vi "Initialise_scan_mirror_positions.vi"(8 "error in (no error)":errorcluster) -> (0 "error out":errorcluster)   [LabVIEW 2012]
uses:
  Custom Controls/scan mode main settings tab.ctl
  GFG/GFGbooleanGet.vi
  <vilib>/DAQmx/create/channels.llb/DAQmx Create Channel (AO-Voltage-Basic).vi
  <vilib>/DAQmx/write.llb/DAQmx Write.vi
  <vilib>/DAQmx/write.llb/DAQmx Write (Analog 1D DBL NChan 1Samp).vi
  GFG/GFGstringGet.vi
  GFG/GFG library.lvlib
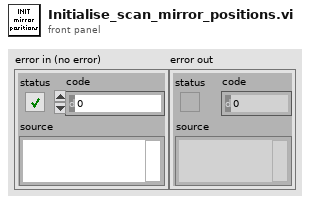
[diagram p1: front panel]
types:
  T1 = typedef "scan mode main settings tab.ctl" = enum32{"2D frame", "2D line scan", "general settings", "Z Stack", "piezo"}
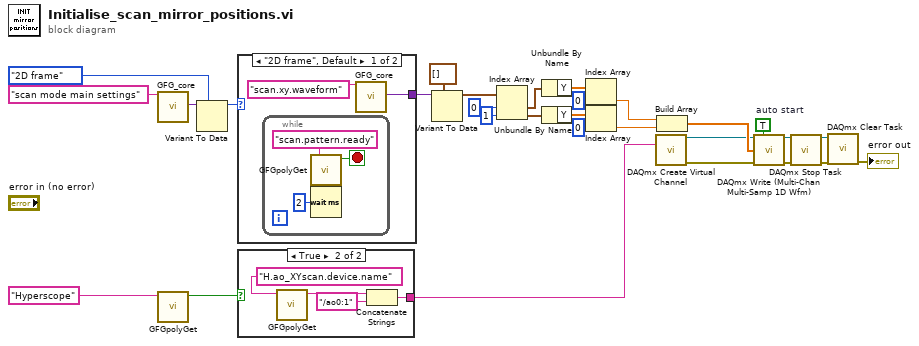
[diagram p0: block diagram]
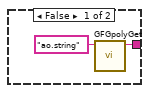
[diagram p2: hidden frame]
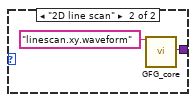
[diagram p3: hidden frame]
diagram:
  w6 = TRUE  # auto start
  n1 = call "GFG_core.vi"("Variable Name in"="scan mode main settings") -> ("Variant Out"=w28:variant)  [unwired: 12 in, 6 out]
  n2 = call-poly "GFGpolyGet.vi"("Variable Name in"="Hyperscope") -> ("Boolean Value OUT"=w13:bool)  [unwired: 9 in, 1 out]
  n3 = Variant To Data(type=scan_mode_main_settings_tab."2D frame" ("scan mode main settings"), Variant=w28) -> (data=w26:T1)  [unwired: 1 in, 1 out]
  n4 = case shown="\"2D frame\", Default" w26 {
    tunnel: [w30 w35] -> w29
    frame "2D frame", Default {
      n5 = while {
        stop <- w33 stop-if-true
        n6 = call-poly "GFGpolyGet.vi"("Variable Name in"="scan.pattern.ready") -> ("Boolean Value OUT"=w33:bool)  [unwired: 9 in, 1 out]
        n7 = Wait (ms)(milliseconds to wait=u32 2) -> ()  [unwired: 1 out]
      }
      n8 = call "GFG_core.vi"("Variable Name in"="scan.xy.waveform") -> ("Variant Out"=w30:variant)  [unwired: 12 in, 6 out]
    }
    frame "2D line scan" {
      n9 = call "GFG_core.vi"("Variable Name in"="linescan.xy.waveform") -> ("Variant Out"=w35:variant)  [unwired: 12 in, 6 out]
    }
  }
  n10 = case shown="True" w13 {
    tunnel: [w37 w39] -> w3
    frame False {
      n11 = call-poly "GFGpolyGet.vi"("Variable Name in"="ao.string" ("name to assign")) -> ("String"=w37:string)  [unwired: 9 in, 1 out]
    }
    frame True {
      n12 = call-poly "GFGpolyGet.vi"("Variable Name in"="H.ao_XYscan.device.name" ("name to assign")) -> ("String"=w41:string)  [unwired: 9 in, 1 out]
      n13 = Concatenate Strings(w41, "/ao0:1" ("string")) -> (w39:string)
    }
  }
  n14 = Variant To Data(type=waveform(dbl)[] [] ("scan.xy.waveform"), Variant=w29) -> (data=w23:waveform(dbl)[])  [unwired: 1 in, 1 out]
  n15 = Index Array(array=w23, index #1=0 ("index"), index #2=1 ("index")) -> (element #1=w20:waveform(dbl), element #2=w19:waveform(dbl))
  n16 = Unbundle By Name(w20) -> ("Y"=w18:dbl[])
  n17 = Unbundle By Name(w19) -> ("Y"=w15:dbl[])
  n18 = Index Array(array=w18, index=0) -> (element=w2:dbl)
  n19 = Index Array(array=w15, index=0) -> (element=w1:dbl)
  n20 = call-poly <vilib>:"DAQmx Create Virtual Channel.vi"("physical channels"=w3) -> ("task out"=w5:refnum<k21>, "error out"=w7:errorcluster)  [unwired: 13 in]
  n21 = Build Array(w2, w1) -> (w12:dbl[])
  n22 = call-poly "DAQmx Write (Multi-Chan Multi-Samp 1D Wfm).vi"("task/channels in"=w5, "auto start"=w6, "data"=w12, "error in"=w7) -> ("task out"=w4:refnum<k21>, "error out"=w8:errorcluster)  [unwired: 9 in, 1 out]
  n23 = call <vilib>:"DAQmx Stop Task.vi"("task/channels in"=w4, "error in"=w8) -> ("task out"=w10:refnum<k21>, "error out"=w9:errorcluster)  [unwired: 12 in]
  n24 = call <vilib>:"DAQmx Clear Task.vi"("task in"=w10, "error in"=w9) -> ("error out"=→"error out":errorcluster)  [unwired: 13 in]
